vi "Get Enabled Remotes.vi"(8 "error in (no error)":errorcluster, 11 "Node Config in":refnum<class "Node Config.lvclass">) -> (0 "error out":errorcluster, 2 "Comms Features":T1, 3 "Node Config out":refnum<class "Node Config.lvclass">)   [LabVIEW 2020, in "VectoConfig.lvlib" / "Node Config.lvclass"]
uses:
  Node Config.lvclass
  Comms Features.ctl
  Node Config.lvclass/Node Config.ctl
  VectoConfig/VectoConfig.lvlib
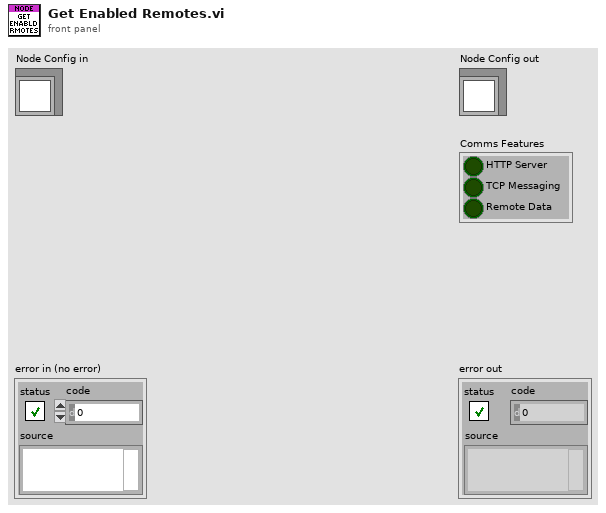
[diagram p1: front panel]
types:
  T1 = typedef "VectoConfig.lvlib/Comms Features.ctl" = cluster{"HTTP Server":bool, "TCP Messaging":bool, "Remote Data":bool}
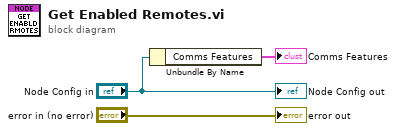
[diagram p0: block diagram]
diagram:
  n1 = Unbundle By Name("Node Config in") -> ("Comms Features"=→"Comms Features":T1)
  "error out" <- "error in (no error)"
  "Node Config out" <- "Node Config in"
